vi "saveDataSN.vi"(8 "error in (no error)":errorcluster, 10 "data":T1, 11 "shot":string) -> (0 "error out":errorcluster)   [LabVIEW 2017]
uses:
  models/dataForSave.ctl
  <vilib>/MDSplus/Library/MDSplus.lvlib
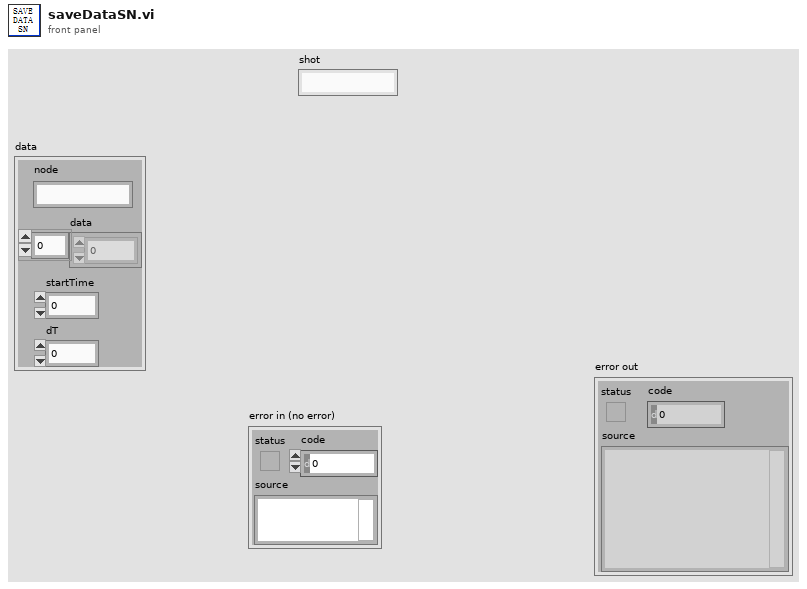
[diagram p1: front panel]
types:
  T1 = typedef "dataForSave.ctl" = cluster{"node":string, "data":dbl[], "startTime":dbl, "dT":dbl}
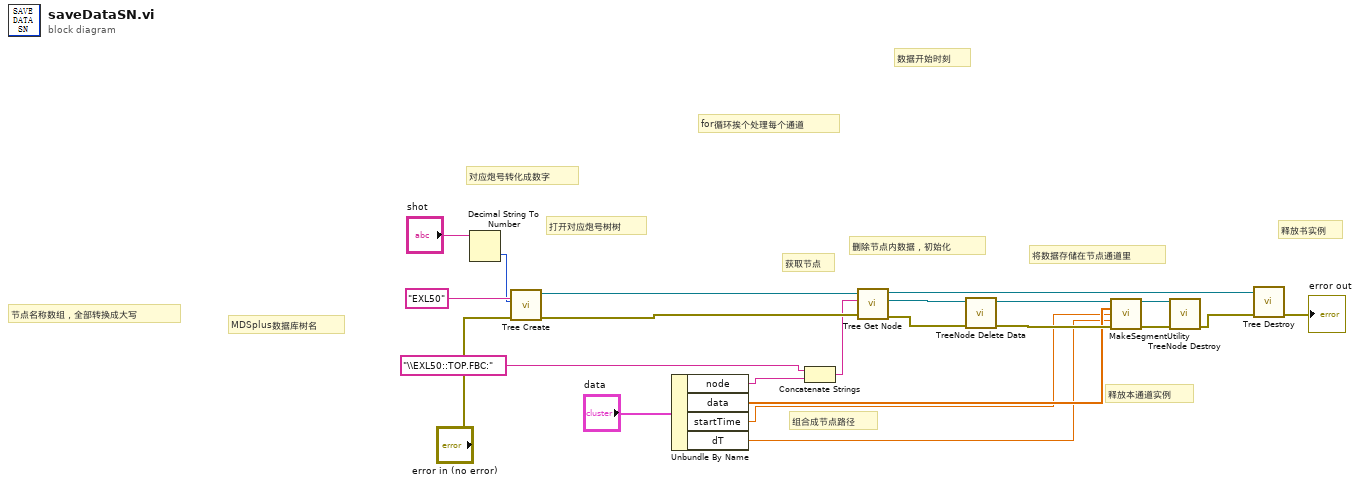
[diagram p0: block diagram]
diagram:
  # "释放本通道实例"
  # "将数据存储在节点通道里"
  # "删除节点内数据，初始化"
  # "获取节点"
  # "组合成节点路径"
  # "数据开始时刻"
  # "for循环挨个处理每个通道"
  # "释放书实例"
  # "打开对应炮号树树"
  # "节点名称数组，全部转换成大写"
  # "MDSplus数据库树名"
  # "对应炮号转化成数字"
  n1 = Decimal String To Number(string="shot") -> (number=w19:i32)  [unwired: 2 in, 1 out]
  n2 = call <vilib>:"Tree Create.vi"("error in (no error)"="error in (no error)", "Shot"=w19, "Name"="EXL50" ("TreeName")) -> ("error out"=w16:errorcluster, "Tree DVR out"=w17:refnum<data-value>)  [unwired: 7 in]
  n3 = Unbundle By Name("data") -> ("node"=w6:string, "data"=w5:dbl[], "startTime"=w4:dbl, "dT"=w3:dbl)
  n4 = Concatenate Strings("\\EXL50::TOP.FBC:" ("字符串"), w6) -> (w11:string)
  n5 = call <vilib>:"Tree Get Node.vi"("error in (no error)"=w16, "Path"=w11, "Tree DVR in"=w17) -> ("error out"=w13:errorcluster, "Node out"=w12:refnum<data-value>, "Tree DVR out"=w2:refnum<data-value>)  [unwired: 6 in]
  n6 = call <vilib>:"TreeNode Delete Data.vi"("error in (no error)"=w13, "TreeNode DVR in"=w12) -> ("error out"=w10:errorcluster, "TreeNode DVR out"=w14:refnum<data-value>)  [unwired: 8 in]
  n7 = call <vilib>:"MakeSegmentUtility.vi"("TreeNode DVR in"=w14, "DBL Array"=w5, "Start time"=w4, "dt"=w3, "error in (no error)"=w10) -> ("TreeNode DVRout"=w9:refnum<data-value>, "error out"=w8:errorcluster)  [unwired: 9 in]
  n8 = call <vilib>:"TreeNode Destroy.vi"("error in (no error)"=w8, "TreeNode DVR in"=w9) -> ("error out"=w1:errorcluster)  [unwired: 9 in]
  n9 = call <vilib>:"Tree Destroy.vi"("error in (no error)"=w1, "Tree DVR in"=w2) -> ("error out"=→"error out":errorcluster)  [unwired: 9 in]
